vi "uA_daq_calculate_All_values_from Sub_chart.vi"(6 "Cursor.Cursor X 2":dbl, 9 "Cursor.Cursor X":dbl, 10 "Value":waveform(sgl), 11 "Sample rate":dbl) -> (1 "Max value":dbl, 2 "Average":dbl, 3 "Delta(s)":sgl, 4 "Min value":dbl)   [LabVIEW 2015]
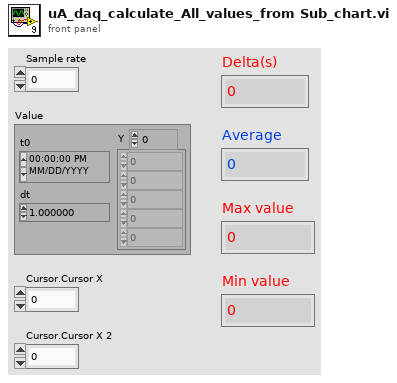
[diagram p1: front panel]
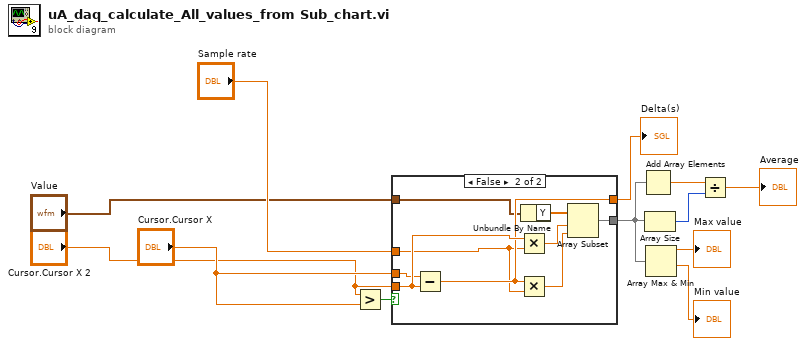
[diagram p0: block diagram]
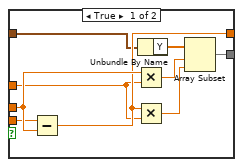
[diagram p2: hidden frame]
diagram:
  n1 = Greater?(x="Cursor.Cursor X 2", y="Cursor.Cursor X") -> (0:w1:bool)
  n2 = case shown="False" w1 {
    tunnel: "Value" -> [w15 w24]
    tunnel: "Cursor.Cursor X 2" -> [w17 w27]
    tunnel: "Cursor.Cursor X" -> [w18 w26]
    tunnel: [w19 w28] -> w8
    tunnel: [w16 w25] -> w7
    tunnel: "Sample rate" -> [w13 w22]
    frame True {
      n3 = Subtract(x=w17, y=w18) -> (x-y=w16:dbl)
      n4 = Multiply(x=w18, y=w13) -> (x*y=w21:dbl)
      n5 = Multiply(x=w16, y=w13) -> (x*y=w20:dbl)
      n6 = Unbundle By Name(w15) -> ("Y"=w14:sgl[])
      n7 = Array Subset(array=w14, index=w21, length=w20) -> (w19:sgl[])
    }
    frame False {
      n8 = Subtract(x=w26, y=w27) -> (x-y=w25:dbl)
      n9 = Multiply(x=w27, y=w22) -> (x*y=w30:dbl)
      n10 = Multiply(x=w25, y=w22) -> (x*y=w29:dbl)
      n11 = Unbundle By Name(w24) -> ("Y"=w23:sgl[])
      n12 = Array Subset(array=w23, index=w30, length=w29) -> (w28:sgl[])
    }
  }
  "Delta(s)" <- w7
  n13 = Add Array Elements(numeric array=w8) -> (sum=w4:sgl)
  n14 = Array Size(array=w8) -> (size(s)=w5:i32)
  n15 = Array Max & Min(array=w8) -> (max value=→"Max value":sgl, min value=→"Min value":sgl)  [unwired: 2 out]
  n16 = Divide(x=w4, y=w5) -> (x/y=→"Average":sgl)
